vi "EditQueryRequest.vi"(8 "error in (no error)":errorcluster) -> (0 "error out":errorcluster)   [LabVIEW 2013, in "main.lvlib"]
uses:
  main.lvlib
  Controls/Enum Variables.ctl
  Controls/Enum Save Action Events.ctl
  <vilib>/xml/Load XML File.vi
  <vilib>/xml/Close Reference(Node).vi
  <vilib>/xml/NI_XML.lvlib
  <resource>/objmgr/DOMUserDefRef.rc
panel:
  in  "EditQueryRequestTable":string[][](table)
  in  "CancelTagsBtn":bool
  in  "SaveTagsBtn":bool
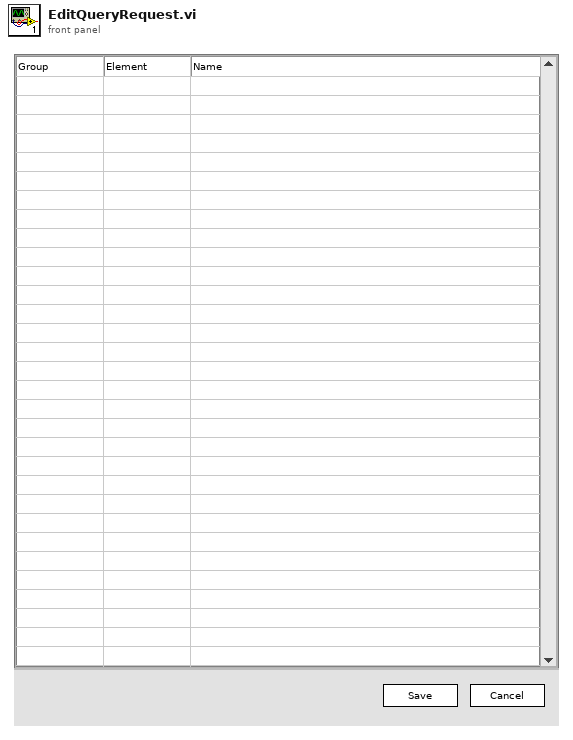
[diagram p1: front panel]
types:
  T1 = typedef "main.lvlib/Enum Variables.ctl" = enum16{"SetAcqFilter", "GetAcqFilter", "Set Filter", "Get Filter", "Set Height", "Get Height", "Set Recorded Height", "Get Recorded Height", "Set Blue Pressure", "Get Blue Pressure", "Set Red Pressure", "Get Red Pressure", "Init", "Reset Pressure", "Set Red Cursors", "Get Red Cursors", "Set Blue Cursors", "Get Blue Cursors", "Set Language", "Get Language", "Set Active Graphs", "Get ActiveGraphs", "Set Method", "Get Method", "Set Encryption", "Get Encryption", "Set ExcelVersion", "Get ExcelVersion", "Set DICOM Avail", "Get DICOM Avail", "Set DICOM Encode", "Get DICOM Encode", "Set JournalExport", "Get JournalExport", "Set Sequence", "Get Sequence", "Set DAQ Connected", "Get DAQ Connected", "Set Current Graph", "Get Current Graph", "Set General Settings", "Get Hyphenation", "Set Arm Calc Method", "Get Arm Calc Method", "Set Dicom Tags", "Get Dicom Tags", "Set BT Serial", "Get BT Serial", "Set BT Accepted Serials", "Get BT Accepted Serials", "Get BT License", "Set BT License"}
  T2 = typedef "main.lvlib/Enum Save Action Events.ctl" = enum16{"LoadReportPath", "SaveReportPath", "Load Graph Path", "Save Graph Path", "LoadDataPath", "SaveDataPath", "Load Template Path", "Save Template Path", "Load PressureFactor", "Save PressureFactor", "Init", "Load Listbox", "Save Listbox", "LoadHospInfo", "SaveHospInfo", "Load DICOM Activation", "Save DICOM Activation", "LoadDICOMInfoWL", "SaveDICOMInfoWL", "LoadDICOMInfoPACS", "SaveDICOMInfoPACS", "Load ArmCalcMethod", "Save ArmCalcMethod", "LoadItemTags", "SaveItemTags", "LoadDICOMEncoding", "SaveDICOMEncoding", "LoadJournalType", "SaveJournalType", "LoadAcqFilterType", "SaveAcqFilterType", "Load Sequence", "Save Sequence", "Load Acquisition Mode", "Save Acquisition Mode", "Load General Settings", "Save General Settings", "Load Language", "Save Language", "Load Dicom Tags", "Save Dicom Tags", "Load BT Serial", "Save BT Serial", "Load BT License", "Save BT License"}
  T3 = typedef "LVRowAndColumnTypeDef.ctl" = cluster{"Row":i32, "Column":i32}
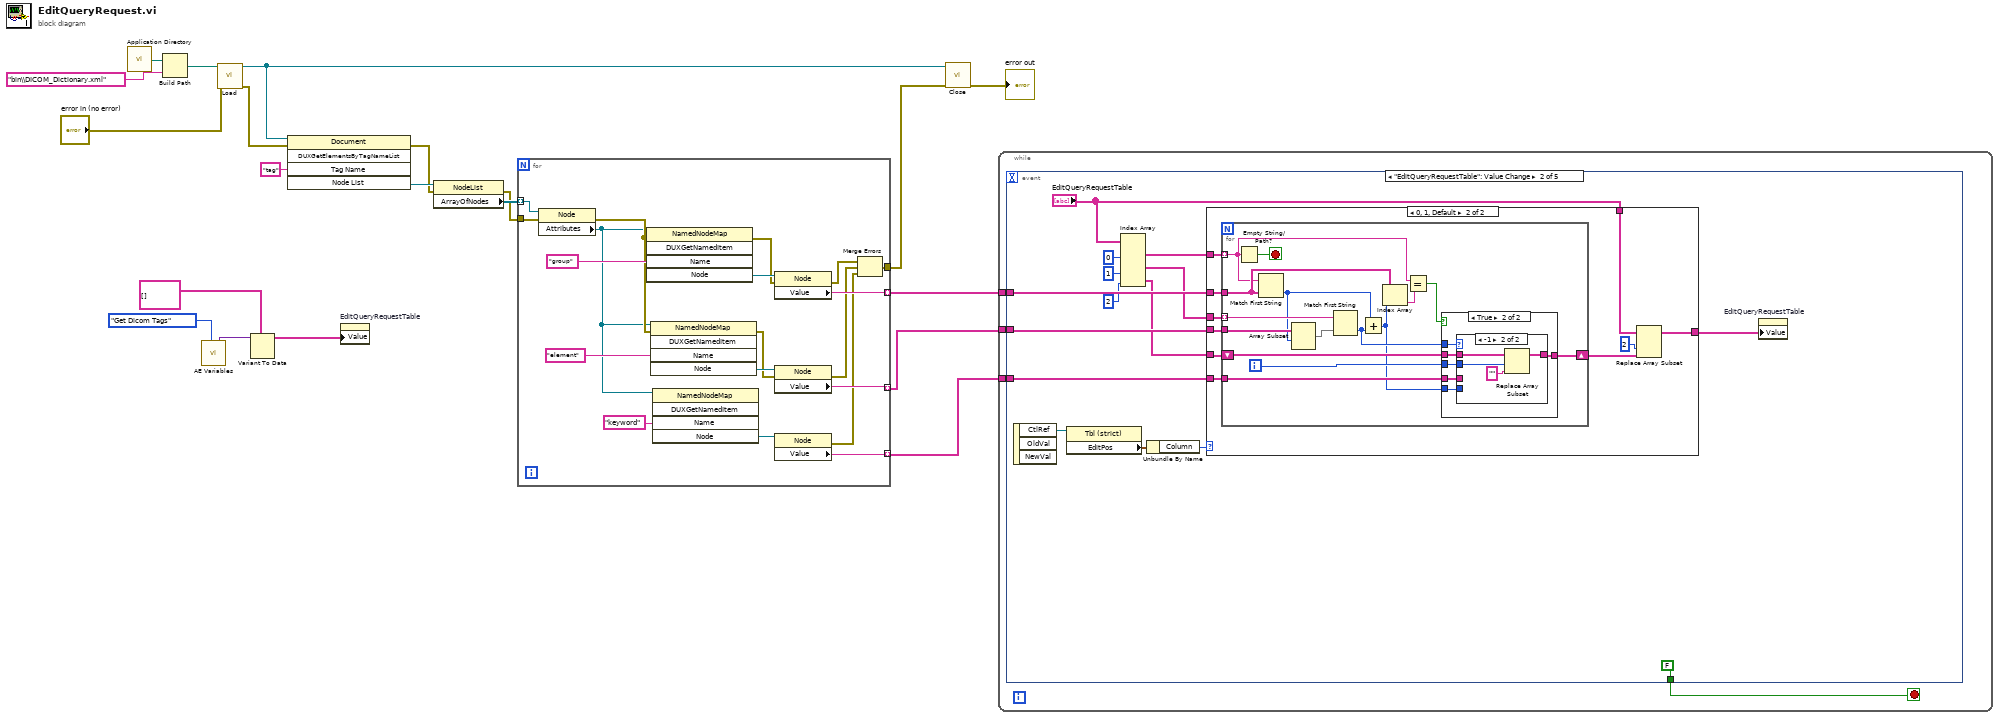
[diagram p0: block diagram]
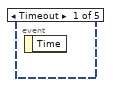
[diagram p2: hidden frame]
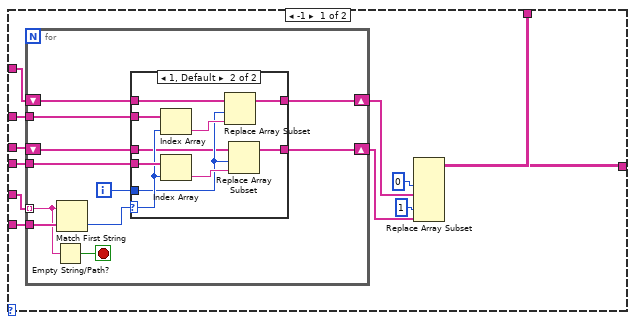
[diagram p3: hidden frame]
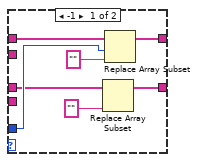
[diagram p4: hidden frame]
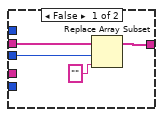
[diagram p5: hidden frame]
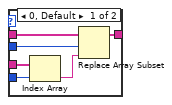
[diagram p6: hidden frame]
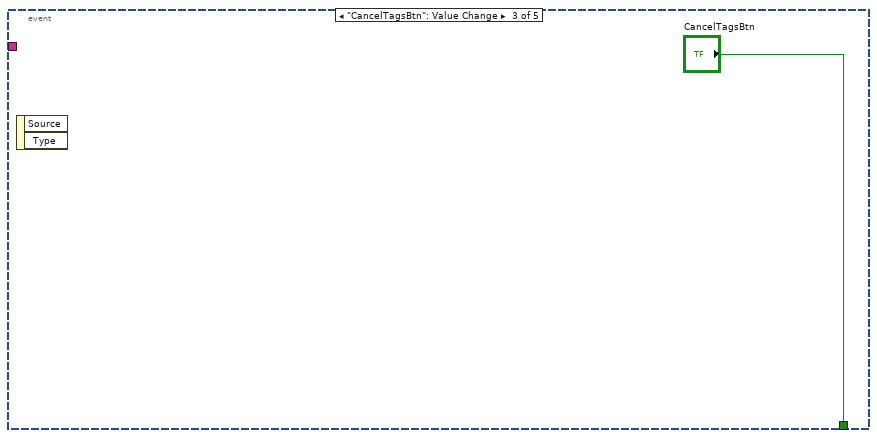
[diagram p7: hidden frame]
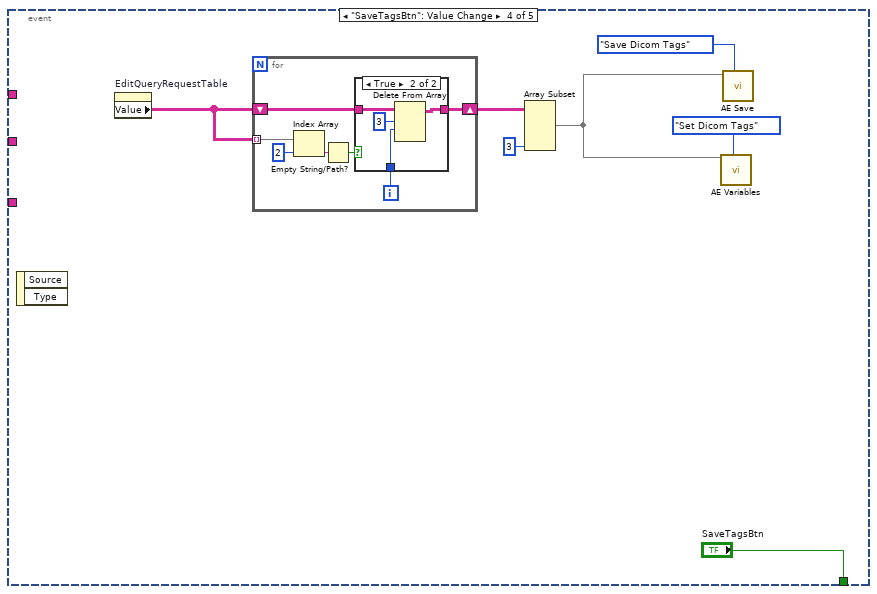
[diagram p8: hidden frame]
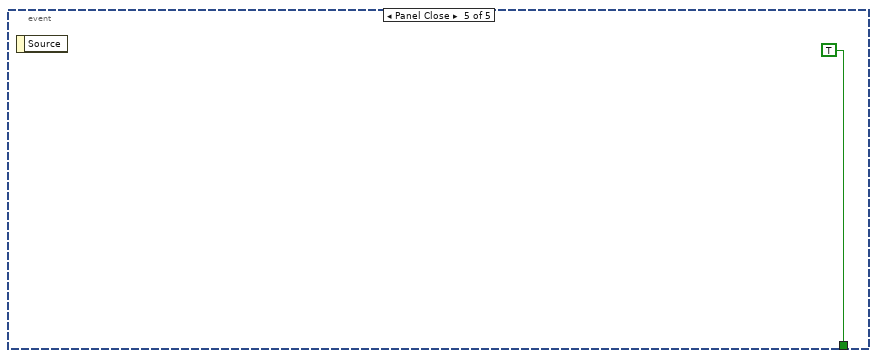
[diagram p10: hidden frame]
diagram:
  n1 = call <vilib>:"Application Directory.vi"() -> ("Application Directory"=w20:path)
  n2 = Build Path(base path=w20, name or relative path="bin\\DICOM_Dictionary.xml") -> (appended path=w18:path)
  n3 = call "AE Variables.vi"("Action"=Enum_Variables."Get Dicom Tags") -> ("Variant"=w3:variant)  [unwired: 11 in, 7 out]
  n4 = call-poly <vilib>:"Load.vi"("path to XML document"=w18, "error in (no error)"="error in (no error)") -> ("DOM document out"=w5:refnum<k20>, "error out"=w12:errorcluster)  [unwired: 11 in, 1 out]
  n5 = Variant To Data(type=string[][] [], Variant=w3) -> (data=w1:string[][])  [unwired: 1 in, 1 out]
  n6 = invoke class="Document" method="DUXGetElementsByTagNameList"(reference=w5, error in=w12, "Tag Name"="tag") -> (error out=w14:errorcluster, "Node List"=w16:refnum<k20>)  [unwired: 2 in, 3 out]
  n7 = property on="EditQueryRequestTable" class="Tbl (strict)"("Value"=w1) -> ()  [unwired: 2 in, 2 out]
  n8 = property class="NodeList"(reference=w16, error in=w14) -> (error out=w13:errorcluster, "ArrayOfNodes"=w15:refnum<k20>[])  [unwired: 1 out]
  n9 = for {
    tunnel: w15 -> [w31] mode=indexing
    tunnel: w13 -> [w39]
    tunnel: [w35] -> w10 mode=indexing
    tunnel: [w32] -> w9 mode=indexing
    tunnel: [w30] -> w8 mode=indexing
    tunnel: [w24] -> w7
    n10 = property class="Node"(reference=w31, error in=w39) -> (error out=w29:errorcluster, "Attributes"=w23:refnum<k20>)  [unwired: 1 out]
    n11 = invoke class="NamedNodeMap" method="DUXGetNamedItem"(reference=w23, error in=w29, "Name"="group") -> (error out=w36:errorcluster, "Node"=w37:refnum<k20>)  [unwired: 2 in, 3 out]
    n12 = invoke class="NamedNodeMap" method="DUXGetNamedItem"(reference=w23, error in=w29, "Name"="element") -> (error out=w28:errorcluster, "Node"=w33:refnum<k20>)  [unwired: 2 in, 3 out]
    n13 = invoke class="NamedNodeMap" method="DUXGetNamedItem"(reference=w23, "Name"="keyword") -> ("Node"=w21:refnum<k20>)  [unwired: 3 in, 4 out]
    n14 = property class="Node"(reference=w37, error in=w36) -> (error out=w25:errorcluster, "Value"=w35:string)  [unwired: 1 out]
    n15 = property class="Node"(reference=w33, error in=w28) -> (error out=w26:errorcluster, "Value"=w32:string)  [unwired: 1 out]
    n16 = property class="Node"(reference=w21) -> (error out=w27:errorcluster, "Value"=w30:string)  [unwired: 1 in, 1 out]
    n17 = Merge Errors(w25, w26, w27) -> (w24:errorcluster)
  }
  n18 = call-poly <vilib>:"Close.vi"("error in (no error)"=w7, "node"=w5) -> ("error out"=→"error out":errorcluster)  [unwired: 7 in]
  n19 = while {
    tunnel: w10 -> [w43]
    tunnel: w9 -> [w42]
    tunnel: w8 -> [w41]
    stop <- w40 stop-if-true
    n20 = event shown="[1] \"EditQueryRequestTable\": Value Change" {
      selector: _ -> [_ _ _ _ _]
      dyn-events: _ -> [_ _ _ _ _]
      timeout: _ -> [_ _ _ _ _]
      tunnel: w43 -> [_ w56 _ _ _]
      tunnel: w42 -> [_ w54 _ _ _]
      tunnel: w41 -> [_ w53 _ _ _]
      tunnel: [_ FALSE "CancelTagsBtn" "SaveTagsBtn" TRUE] -> w40
      event Timeout {
        n21 = event-data() -> ()  [unwired: 1 in, 1 out]
      }
      event "EditQueryRequestTable": Value Change {
        n22 = event-data() -> ("CtlRef"=w49:refnum<vi>)  [unwired: 1 in, 2 out]
        n23 = property class="Tbl (strict)"(reference=w49) -> ("EditPos"=w48:T3)  [unwired: 1 in, 2 out]
        n24 = Index Array(array="EditQueryRequestTable", index (col) #1=0 ("disabled index (col)"), index (col) #2=1 ("index (col)"), index (col) #3=2 ("index (col)")) -> (element #1=w57:string[], element #2=w55:string[], element #3=w46:string[])  [unwired: 3 in]
        n25 = Unbundle By Name(w48) -> ("Column"=w47:i32)
        n26 = case shown="0, 1, Default" w47 {
          tunnel: w57 -> [w66 w108]
          tunnel: w56 -> [w68 w107]
          tunnel: w55 -> [w65 w106]
          tunnel: w54 -> [w69 w105]
          tunnel: w53 -> [w70 w104]
          tunnel: w46 -> [w67 w103]
          tunnel: [w59 w101] -> w44
          tunnel: "EditQueryRequestTable" -> [w60 w102]
          frame -1 {
            n27 = for {
              tunnel: w68 -> [w78]
              tunnel: w69 -> [w79]
              tunnel: w70 -> [w80]
              tunnel: w67 -> [w77] mode=indexing
              shift-right: [w74] -> w63
              shift-left: w66 -> [w73]
              shift-right: [w72] -> w61
              shift-left: w65 -> [w71]
              i -> [w75]
              stop <- w81 stop-if-true
              n28 = Empty String/Path?(string/path=w77) -> (empty?=w81:bool)
              n29 = Match First String(2:w80, 3:w77) -> (0:w76:i32)  [unwired: 1 out]
              n30 = case shown="1, Default" w76 {
                selector: w76 -> [_ w96]
                tunnel: w79 -> [_ w98]
                tunnel: w78 -> [_ w97]
                tunnel: w75 -> [w86 w91]
                tunnel: [w85 w94] -> w74
                tunnel: w73 -> [w88 w93]
                tunnel: [w83 w90] -> w72
                tunnel: w71 -> [w82 w89]
                frame -1 {
                  n31 = Replace Array Subset(array=w82, new element="" ("new element/subarray")) -> (w83:string[])  [unwired: 1 in]
                  n32 = Replace Array Subset(array=w88, new element="" ("new element/subarray"), index=w86) -> (w85:string[])
                }
                frame 1, Default {
                  n33 = Index Array(array=w97, index=w96) -> (element=w95:string)
                  n34 = Index Array(array=w98, index=w96) -> (element=w92:string)
                  n35 = Replace Array Subset(array=w93, new element=w95, index=w91) -> (w94:string[])
                  n36 = Replace Array Subset(array=w89, new element=w92, index=w91) -> (w90:string[])
                }
              }
            }
            n37 = Replace Array Subset(array=w60, new element #1=w63, index (col) #1=0 ("disabled index (col)"), new element #2=w61, index (col) #2=1 ("disabled index (col)")) -> (w59:string[][])  [unwired: 2 in]
          }
          frame 0, 1, Default {
            n38 = for {
              tunnel: w108 -> [w109] mode=indexing
              tunnel: w107 -> [w112]
              tunnel: w106 -> [w122] mode=indexing
              tunnel: w105 -> [w121]
              tunnel: w104 -> [w118]
              shift-right: [w115] -> w99
              shift-left: w103 -> [w117]
              i -> [w116]
              stop <- w123 stop-if-true
              n39 = Empty String/Path?(string/path=w109) -> (empty?=w123:bool)
              n40 = Match First String(2:w112, 3:w109) -> (0:w119:i32)  [unwired: 1 out]
              n41 = Array Subset(array=w121, index=w119) -> (w120:string[])  [unwired: 1 in]
              n42 = Match First String(2:w120, 3:w122) -> (0:w114:i32)  [unwired: 1 out]
              n43 = Add(x=w119, y=w114) -> (x+y=w113:i32)
              n44 = Index Array(array=w112, index=w113) -> (element=w111:string)
              n45 = Equal?(x=w109, y=w111) -> (x = y?=w110:bool)
              n46 = case shown="True" w110 {
                tunnel: w118 -> [_ w133]
                tunnel: w117 -> [w125 w132]
                tunnel: w116 -> [w124 w131]
                tunnel: [w126 w130] -> w115
                tunnel: w114 -> [_ w129]
                tunnel: w113 -> [_ w128]
                frame False {
                  n47 = Replace Array Subset(array=w125, new element="" ("new element/subarray"), index=w124) -> (w126:string[])
                }
                frame True {
                  n48 = case shown="-1" w129 {
                    tunnel: w133 -> [w139 _]
                    tunnel: w128 -> [w138 _]
                    tunnel: w132 -> [w136 w142]
                    tunnel: w131 -> [w135 w141]
                    tunnel: [w134 w143] -> w130
                    frame 0, Default {
                      n49 = Index Array(array=w139, index=w138) -> (element=w137:string)
                      n50 = Replace Array Subset(array=w136, new element=w137, index=w135) -> (w134:string[])
                    }
                    frame -1 {
                      n51 = Replace Array Subset(array=w142, new element="" ("new element/subarray"), index=w141) -> (w143:string[])
                    }
                  }
                }
              }
            }
            n52 = Replace Array Subset(array=w102, new element=w99, index (col)=2 ("disabled index (col)")) -> (w101:string[][])  [unwired: 1 in]
          }
        }
        n53 = property on="EditQueryRequestTable" class="Tbl (strict)"("Value"=w44) -> ()  [unwired: 2 in, 2 out]
      }
      event "CancelTagsBtn": Value Change {
        n54 = event-data() -> ()  [unwired: 1 in, 2 out]
      }
      event "SaveTagsBtn": Value Change {
        n55 = event-data() -> ()  [unwired: 1 in, 2 out]
        n56 = property on="EditQueryRequestTable" class="Tbl (strict)"() -> ("Value"=w145:string[][])  [unwired: 2 in, 2 out]
        n57 = for {
          shift-right: [w158] -> w146
          shift-left: w145 -> [w156]
          tunnel: w145 -> [w155] mode=indexing
          i -> [w157]
          n58 = Index Array(array=w155, index=2) -> (element=w154:string)
          n59 = Empty String/Path?(string/path=w154) -> (empty?=w152:bool)
          n60 = case shown="True" w152 {
            tunnel: w156 -> [w159 w162]
            tunnel: [w159 w163] -> w158
            tunnel: w157 -> [_ w161]
            frame False {
            }
            frame True {
              n61 = Delete From Array(array=w162, length=3, index (row)=w161) -> (array with subset deleted=w163:string[][])  [unwired: 1 in, 1 out]
            }
          }
        }
        n62 = Array Subset(array=w146, length (col)=3 ("length")) -> (w148:string[][])  [unwired: 3 in]
        n63 = call "AE Variables.vi"("VariantIn"=w148, "Action"=Enum_Variables."Set Dicom Tags") -> ()  [unwired: 10 in, 8 out]
        n64 = call "AE Save.vi"("Variant In"=w148, "Action"=Enum_Save_Action_Events."Save Dicom Tags") -> ()  [unwired: 7 in, 2 out]
      }
      event Panel Close {
        n65 = event-data() -> ()  [unwired: 1 in, 1 out]
      }
    }
  }
